vi "Generate Time Array.vi"(4 "Data rate (Hz)":dbl, 6 "Data":dbl[](array[numeric])) -> (1 "Time Array (s)":dbl[](array[numeric]))   [LabVIEW 2014]
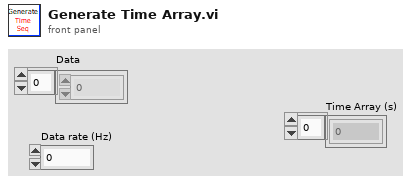
[diagram p1: front panel]
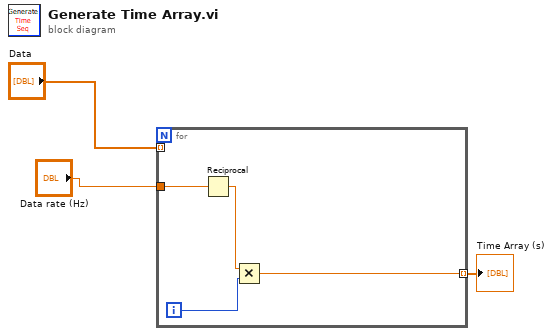
[diagram p0: block diagram]
diagram:
  n1 = for {
    tunnel: "Data rate (Hz)" -> [w5]
    tunnel: [w4] -> w2 mode=indexing
    tunnel: "Data" -> [_] mode=indexing
    i -> [w7]
    n2 = Reciprocal(x=w5) -> (1/x=w6:dbl)
    n3 = Multiply(x=w6, y=w7) -> (x*y=w4:dbl)
  }
  "Time Array (s)" <- w2
